vi "004JohnsDayANs.vi"() -> ()   [LabVIEW 2010]
panel:
  out "johnsLightIsOn":bool
  in  "Time of day":dbl(slide) scale=0.0..24.0
  # "[Johns light]"
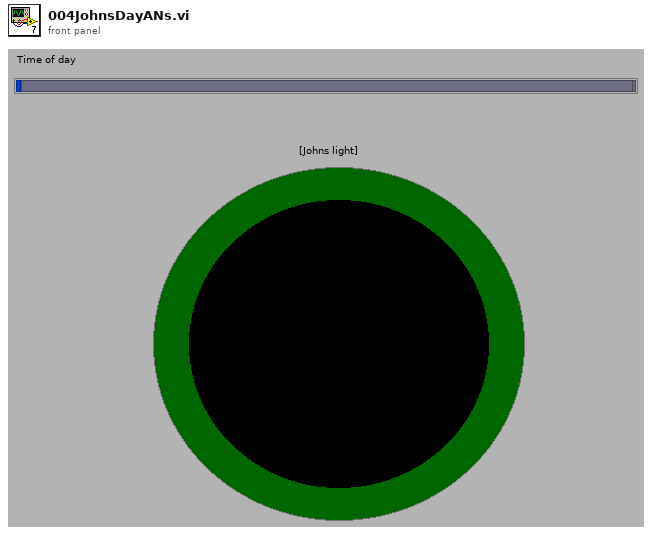
[diagram p1: front panel]
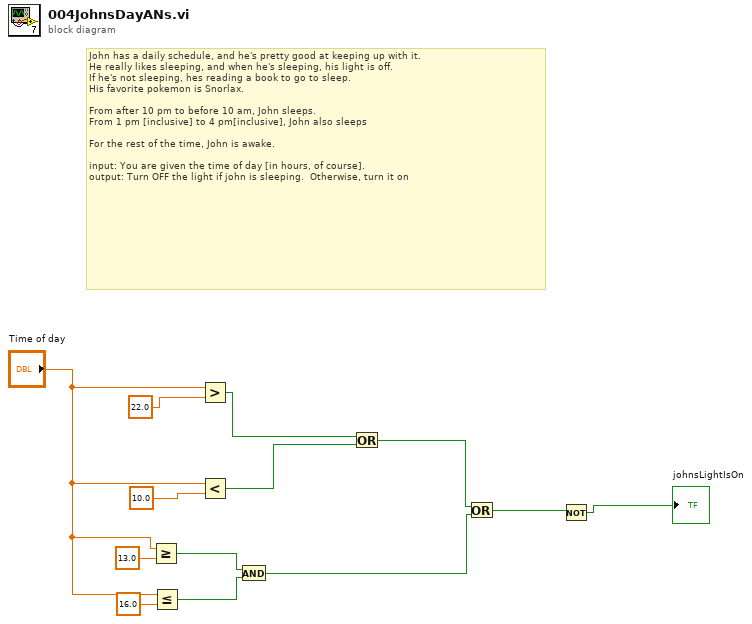
[diagram p0: block diagram]
diagram:
  # "John has a daily schedule, and he's pretty good at keeping up with it.\nHe really likes sleeping, and when he's sleeping, his light is off.  \nIf he's not sleeping, hes reading a book to go to sleep.\nHis favorite pokemon is Snorlax.\n\nFrom after 10 pm to before 10 am, John sleeps.\nFrom 1 pm [inclusive] to 4 pm[inclusive], John also sleeps\n\nFor the rest of the time, John is awake.\n\ninput: You are given the time of day [in hours, of course].  \noutput: Turn OFF the light if john is sleeping.  Otherwise, turn it on"
  n1 = Greater Or Equal?(x="Time of day", y=13.0) -> (x >= y?=w6:bool)
  n2 = Less Or Equal?(x="Time of day", y=16.0) -> (x <= y?=w5:bool)
  n3 = Greater?(x="Time of day", y=22.0) -> (0:w12:bool)
  n4 = Less?(x="Time of day", y=10.0) -> (x < y?=w10:bool)
  n5 = And(x=w6, y=w5) -> (x .and. y?=w3:bool)
  n6 = Or(x=w12, y=w10) -> (x .or. y?=w4:bool)
  n7 = Or(x=w4, y=w3) -> (x .or. y?=w2:bool)
  n8 = Not(x=w2) -> (.not. x?=→"johnsLightIsOn":bool)
